vi "Equi-Ripple LowPass (CDB).vi"(0 "# of taps":i32=32, 1 "pass freq":dbl=0.2 format="%0.2f", 2 "stop freq":dbl=0.25 format="%0.2f", 3 "sampling freq: fs":dbl=1.0 format="%0.2f", 5 "X":cdb[](array[numeric])) -> (4 "error":i32, 7 "Filtered X":cdb[](array[numeric]))   [LabVIEW 2024, in "NI_AALBase.lvlib"]
doc: "<p>Generates a lowpass FIR filter with equi-ripple characteristics using the Parks-McClellan algorithm and the <strong># of taps</strong>, <strong>pass freq</strong>, <strong>stop freq</strong>, and <strong>sampling freq: fs</strong>. The Equi-Ripple LowPass VI then applies a linear-phase, lowpass filter to the input sequence <strong>X</strong> using the <a href=\"nihelplauncher://docs/csh?context=lvcore_lvanls_convolution\">Convolution</a> VI to obtain <strong>Filtered X</strong>. Wire data to the <strong>X</strong> input to determine the polymorphic instance to use or <a href=\"nihelplauncher://docs/csh?context=lvcore_lvhowto_selectingdefaultinstpolyvi\">manually select</a> the instance.</p>"
uses:
  NI_AALBase.lvlib
  1D Convolution (DBL).vi
  NI_AALPro.lvlib
panel:
  # "Equi-Ripple\n Lowpass FIR Filter"
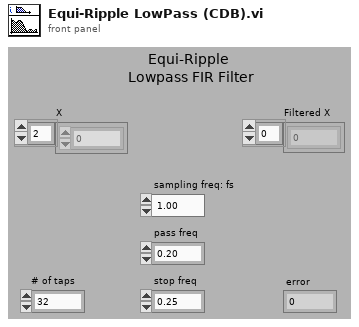
[diagram p1: front panel]
types:
  T1 = cluster{"Amplitude":dbl, "DC":dbl, "pass freq":dbl, "Weight":dbl}
  T2 = cluster{"Amplitude":dbl, "stop freq":dbl, dbl, "Weight":dbl}
  T3 = cluster{"Amplitude":dbl, "stop freq":dbl, "pass freq":dbl, "Weight":dbl}[]
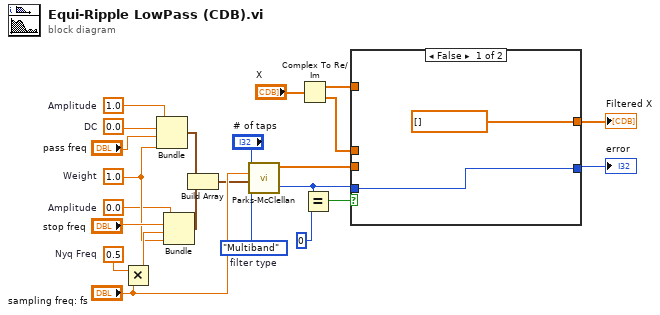
[diagram p0: block diagram]
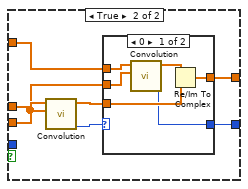
[diagram p2: hidden frame]
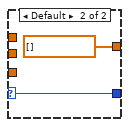
[diagram p3: hidden frame]
diagram:
  w3 = enum32{"Multiband", "Differentiator", "Hilbert"}."Multiband"  # filter type
  w20 = 0.5  # Nyq Freq
  w4 = 0.0  # Amplitude
  w5 = 1.0  # Weight
  w23 = 0.0  # DC
  w6 = 1.0  # Amplitude
  n1 = Multiply(x=w20, y="sampling freq: fs") -> (x*y=w19:dbl)
  n2 = Bundle("Amplitude"=w6, "DC"=w23, "pass freq"="pass freq", "Weight"=w5) -> (w18:T1)  [unwired: 1 in]
  n3 = Bundle("Amplitude"=w4, "stop freq"="stop freq", w19, "Weight"=w5) -> (w17:T2)  [unwired: 1 in]
  n4 = Build Array(w18, w17) -> (w10:T3)
  n5 = call "Parks-McClellan.vi"("filter type"=w3, "Band Parameters"=w10, "sampling freq: fs"="sampling freq: fs", "# of taps"="# of taps") -> ("error"=w7:i32, "h"=w9:dbl[])  [unwired: 1 out]
  n6 = Complex To Re/Im(x + iy="X") -> (x=w1:dbl[], y=w2:dbl[])
  n7 = Equal?(x=w7, y=0) -> (x = y?=w16:bool)
  n8 = case shown="False" w16 {
    tunnel: w7 -> [w25 _]
    tunnel: [w25 w26] -> w15
    tunnel: [cdb[] [] ("empty array") w28] -> w14
    tunnel: w2 -> [_ w32]
    tunnel: w9 -> [_ w29]
    tunnel: w1 -> [_ w30]
    frame False {
    }
    frame True {
      n9 = call-poly "Convolution.vi"("Y"=w29, "X"=w32) -> ("error"=w31:i32, "X * Y"=w27:dbl[])  [unwired: 8 in]
      n10 = case shown="0" w31 {
        selector: w31 -> [_ w39]
        tunnel: w30 -> [w38 _]
        tunnel: w29 -> [w37 _]
        tunnel: [w35 cdb[] [] ("empty array")] -> w28
        tunnel: w27 -> [w36 _]
        tunnel: [w34 w39] -> w26
        frame 0 {
          n11 = call-poly "Convolution.vi"("Y"=w37, "X"=w38) -> ("error"=w34:i32, "X * Y"=w33:dbl[])  [unwired: 8 in]
          n12 = Re/Im To Complex(1:w36, 2:w33) -> (0:w35:cdb[])
        }
        frame Default {
        }
      }
    }
  }
  "Filtered X" <- w14
  "error" <- w15
